vi "Changed UI.vi"(11 "Process in":refnum<class "Process.lvclass">) -> (0 "error out":errorcluster, 3 "Process out":refnum<class "Process.lvclass">)   [LabVIEW 2021, in "Process.lvlib" / "Process.lvclass"]
uses:
  Process.lvclass
  Process.lvclass/Process.ctl
  AAM/AAM/Self Actor/Self Actor.lvclass
  AAM/AAM/Msg/Msg.lvclass
  AAM/AAM/Self Actor/Self Msg Send.vi
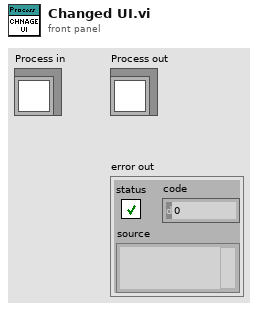
[diagram p1: front panel]
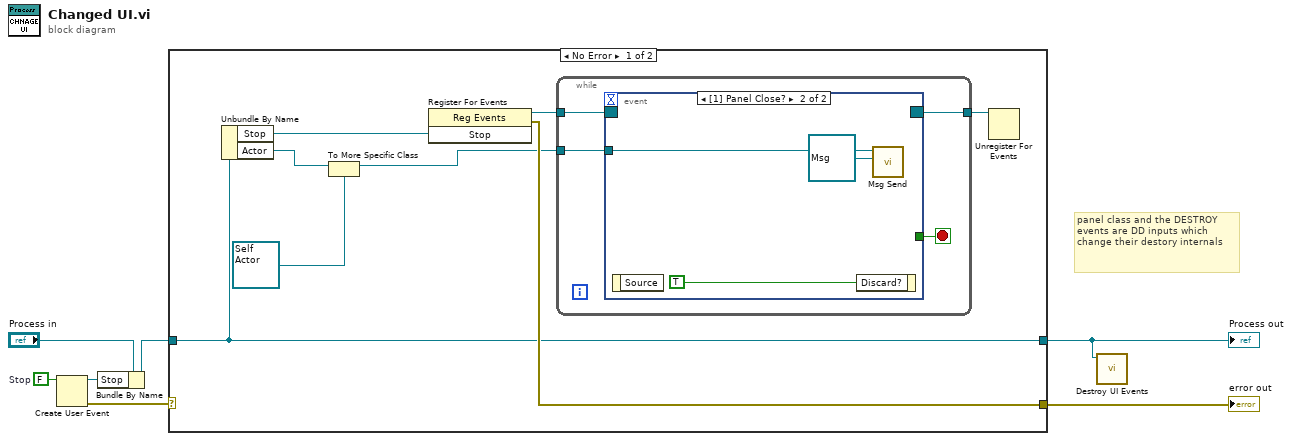
[diagram p0: block diagram]
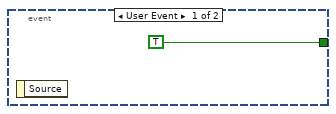
[diagram p2: hidden frame]
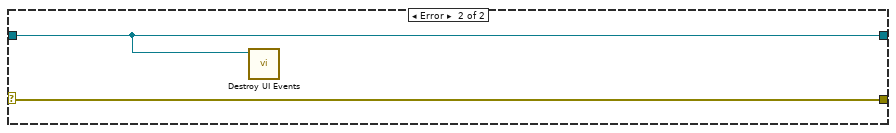
[diagram p3: hidden frame]
diagram:
  w5 = FALSE  # Stop
  # "panel class and the DESTROY events are DD inputs which change their destory internals"
  n1 = Create User Event(user event datatype=w5) -> (user event=w6:refnum<user-event>, error out=w2:errorcluster)  [unwired: 1 in]
  n2 = Bundle By Name(cluster="Process in", "Stop"=w6) -> (w3:refnum<class "Process.lvclass">)
  n3 = case shown="No Error" w2 {
    selector: w2 -> [_ w25]
    tunnel: [w13 w25] -> w4
    tunnel: w3 -> [w10 w24]
    tunnel: [w10 w24] -> w1
    frame No Error {
      n4 = Unbundle By Name(w10) -> ("Stop"=w12:refnum<user-event>, "Actor"=w11:refnum<class "Actor.lvclass">)
      n5 = To More Specific Class(target class=refnum<class "Self Actor.lvclass"> refnum ("AAM.lvlib:Self Actor.lvclass"), reference=w11) -> (specific class reference=w9:refnum<class "Self Actor.lvclass">)  [unwired: 1 in, 1 out]
      n6 = register-events ("Main Register for Events")(w12) -> (reference out=w15:refnum<event-registration>, error out=w13:errorcluster)  [unwired: 2 in]
      n7 = while {
        tunnel: w15 -> [w19]
        tunnel: [w17] -> w14
        tunnel: w9 -> [w16]
        stop <- w18 stop-if-true
        n8 = event "UI Events" shown="[1] Panel Close?" {
          selector: w19 -> [_ _]
          dyn-events: [_ _] -> w17
          timeout: _ -> [_ _]
          tunnel: [TRUE _] -> w18
          tunnel: w16 -> [_ w22]
          event User Event {
            n9 = event-data() -> ()  [unwired: 1 in, 1 out]
          }
          event Panel Close? {
            n10 = event-data() -> ()  [unwired: 1 in, 1 out]
            n11 = event-data("Discard?"=TRUE) -> ()  [unwired: 1 in, 1 out]
            n12 = call-poly "Msg Send.vi"("Msg"=refnum<class "Msg.lvclass"> refnum, "Self Actor in"=w22) -> ()  [unwired: 9 in, 1 out]
          }
        }
      }
      n13 = Unregister For Events(event registration refnum=w14) -> ()  [unwired: 1 in, 1 out]
    }
    frame Error {
      n14 = call "Destroy UI Events.vi"("Process in"=w24) -> ()  [unwired: 11 in]
    }
  }
  "error out" <- w4
  "Process out" <- w1
  n15 = call "Destroy UI Events.vi"("Process in"=w1) -> ()  [unwired: 11 in]
